vi "Create_Raw_data_file.vi"(4 "No of averages":i32=1, 5 "End time":dbl, 6 "Start time":dbl, 7 "Setup filename":string) -> (0 "Error String":string, 1 "Values":string[][](array[string]), 2 "Header Comments":string[](array[string]), 3 "Column headers":string[](array[string]))   [LabVIEW 2010]
uses:
  Controls/Post_Process.ctl
  Globals/Preference_global.vi
  Globals/Meas_global.vi
  Globals/Constants_global.vi
  Globals/Trav_pos_global.vi
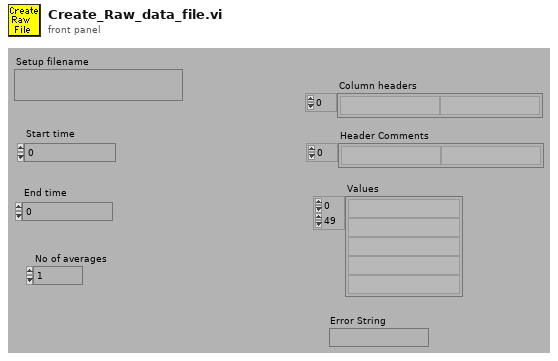
[diagram p1: front panel]
types:
  T1 = typedef "Post_Process.ctl" = enum16{"Take New Data", "Post Process Raw Data File"}
  T2 = typedef "Server_Comms.ctl" = enum16{"Server Link Healthy", "Do Not Link To Server"}
  T3 = typedef "Traverse_cluster.ctl" = cluster{"Start X":dbl, "Start Y":dbl, "Start Z":dbl, "End X":dbl, "End Y":dbl, "End Z":dbl, "No. of pts.":i32, "Spacing":T4, "Filename":path, "Tunnel Speed":dbl, "Averaging time (min)":dbl, "Extra Commands":string, "Specific Arguments":string, "Emission Rate (l/min)":dbl, "Trace Gas Concentration (%)":dbl, "Density Ratio":string, "Comments":string, "Row No":i32, "Row Type Selector":T5, "Completion time":string, "Row Duration (mins)":dbl, "No. of Valid pts.":i32, "Meas Setup File":string}
  T4 = typedef "Spacing.ctl" = enum16{"Linear", "Log", "Gauss", "Specified", "N/A"}
  T5 = typedef "Multi_run_mode.ctl" = enum16{"Move Traverse Only", "Set Tunnel Speed Only", "Set Source Only", "Set Measurement Conditions", "Single Measurement", "Vertical Profile", "Lateral Profile", "Longitudinal Profile", "Explore Volume", "Multi-Axis Profile", "Auto Calibrate", "Meas Fast FID Bkgnd", "Check Beam Power", "Scanning Valve Measurement", "Run VI Named:", "Set ADAM Ch", "Wait (minutes)", "Send Message", "Synchronize With:", "Fall Back to this Row", "Turn Off Row Repeating", "Blank Row"}
  T6 = cluster{"Name":string, "X":dbl, "Y":dbl, "Z":dbl}[]
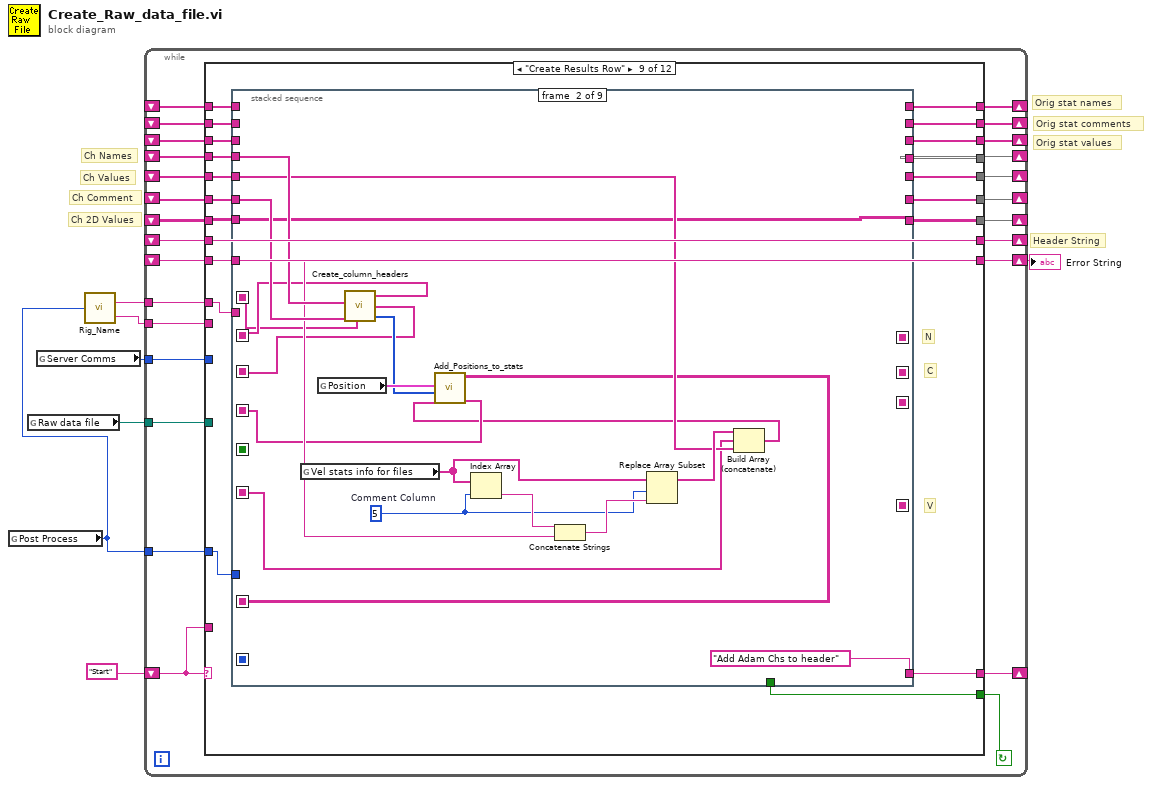
[diagram p0: block diagram]
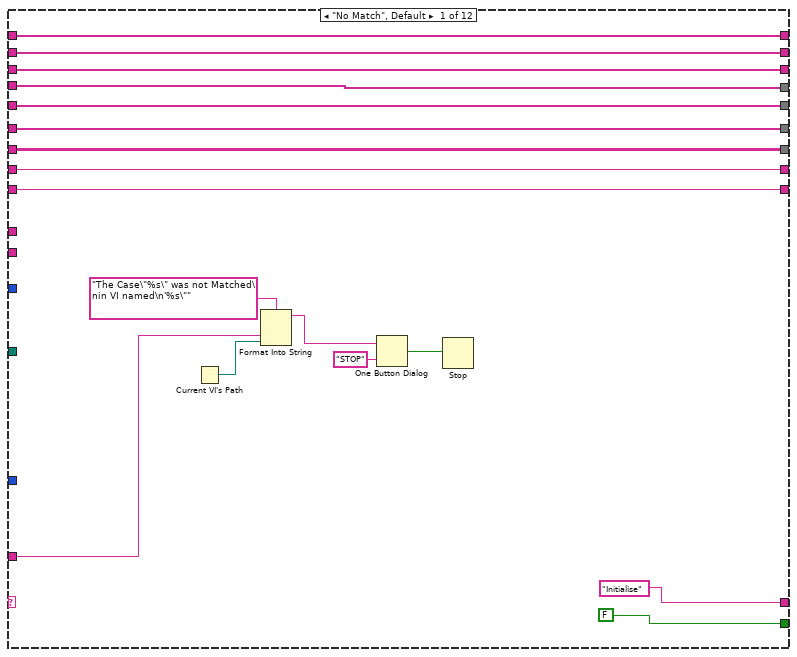
[diagram p2: hidden frame]
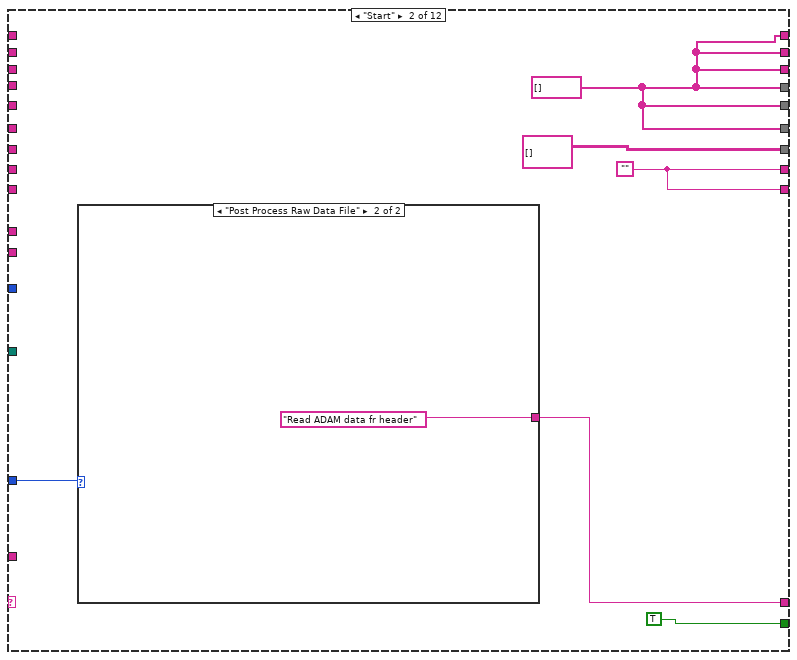
[diagram p3: hidden frame]
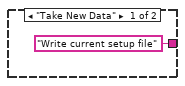
[diagram p4: hidden frame]
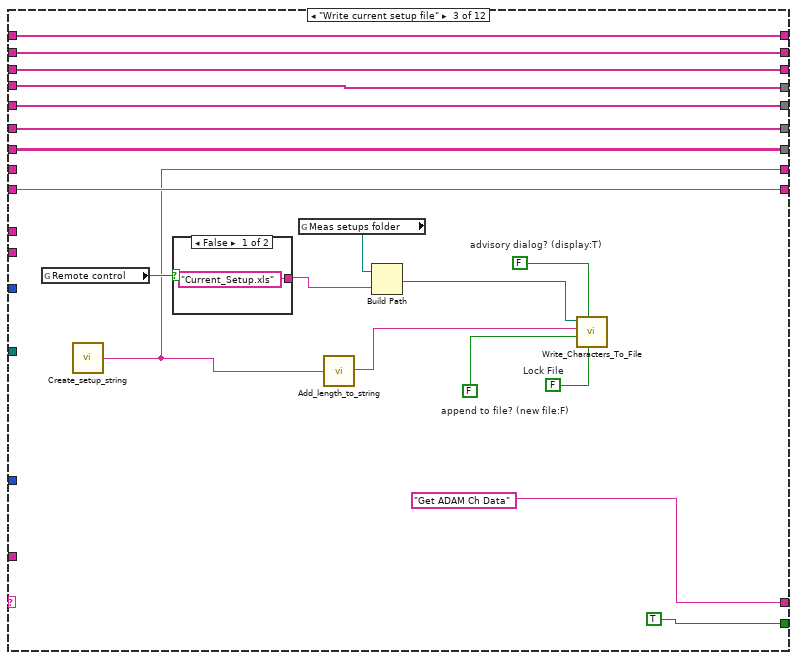
[diagram p5: hidden frame]
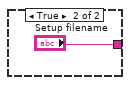
[diagram p6: hidden frame]
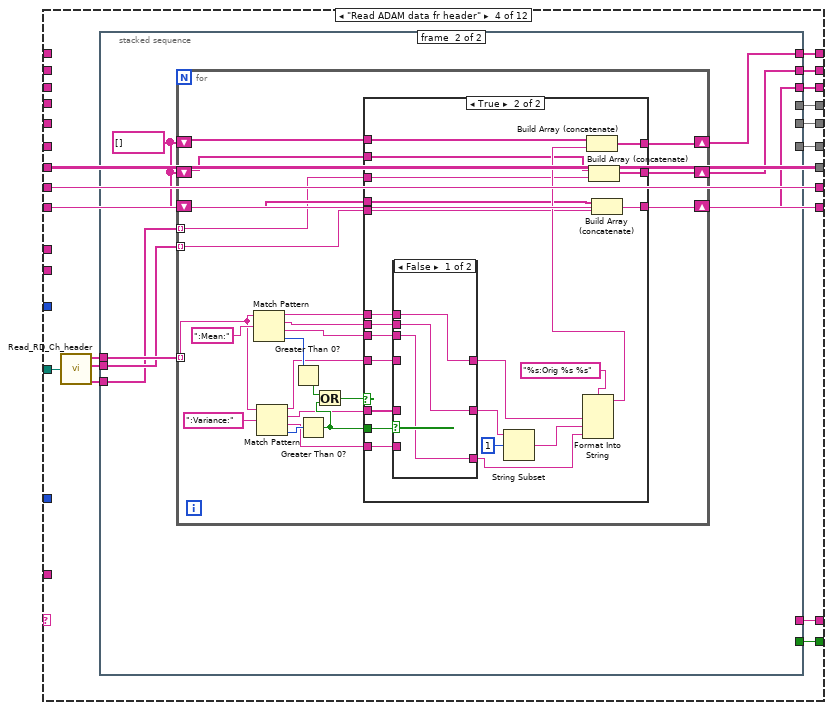
[diagram p7: hidden frame]
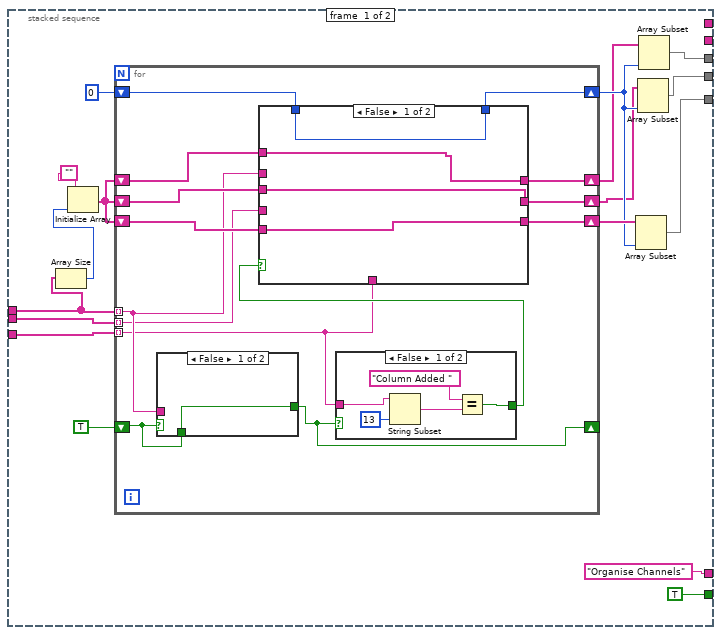
[diagram p8: hidden frame]
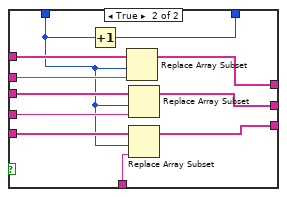
[diagram p9: hidden frame]
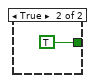
[diagram p10: hidden frame]
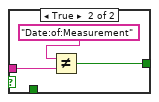
[diagram p11: hidden frame]
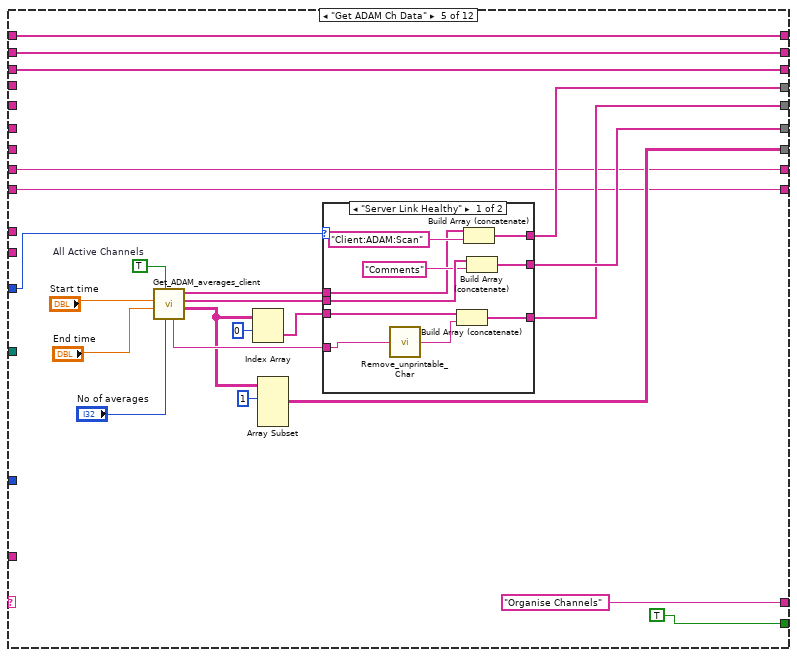
[diagram p14: hidden frame]
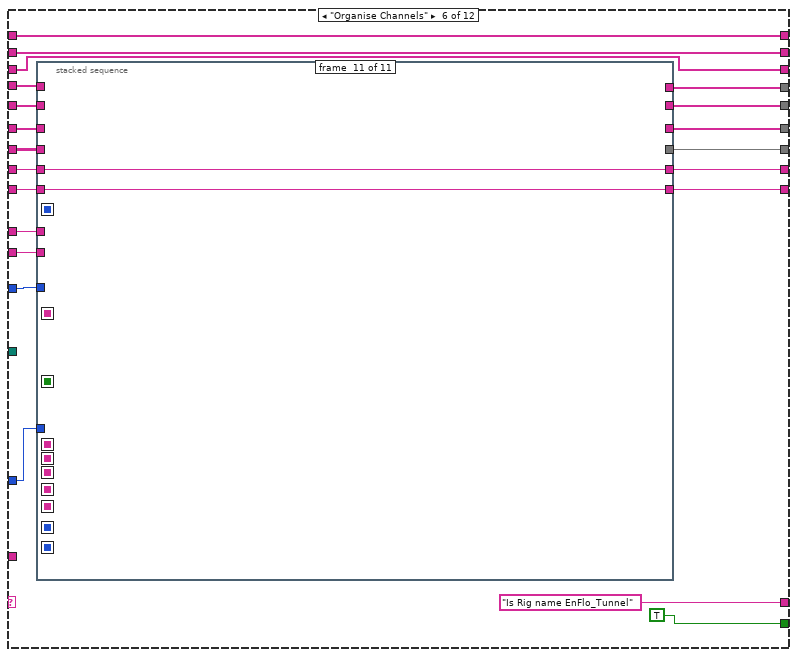
[diagram p16: hidden frame]
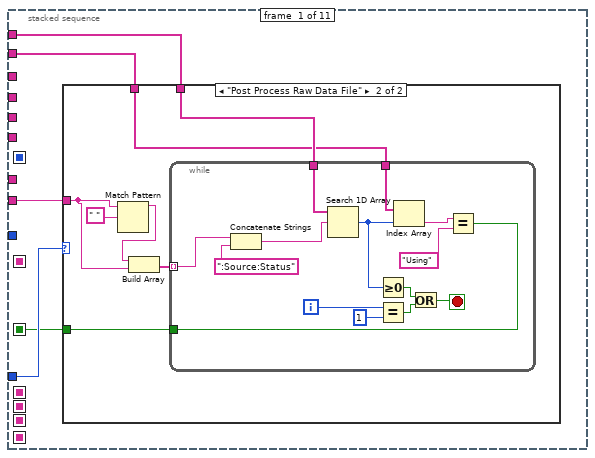
[diagram p17: hidden frame]
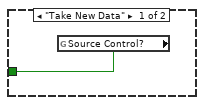
[diagram p18: hidden frame]
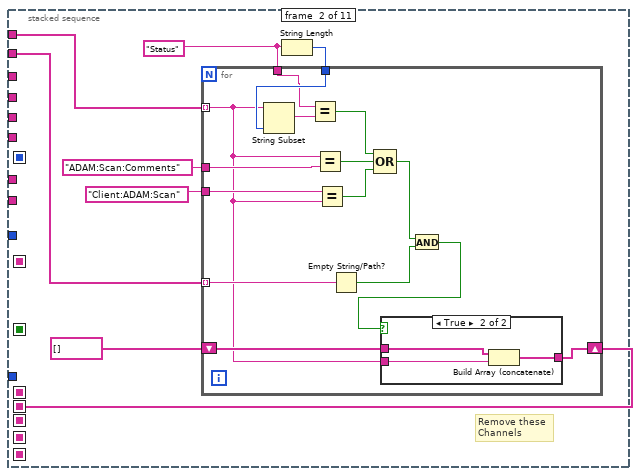
[diagram p19: hidden frame]
diagram:
  # "Orig stat values"
  # "Orig stat comments"
  # "Orig stat names"
  # "Header String"
  # "Ch 2D Values"
  # "Ch Comment"
  # "Ch Values"
  # "Ch Names"
  n1 = global read "Meas_global.vi" "Post Process"() -> (w3:T1)
  n2 = global read "Meas_global.vi" "Raw data file"() -> (w6:path)
  n3 = global read "Preference_global.vi" "Server Comms"() -> (w5:T2)
  n4 = call "Rig_Name.vi"("Post Process"=w3) -> ("Rig Setup before dash"=w2:string, "Hard Disk name"=w1:string)
  n5 = while {
    tunnel: w5 -> [w16]
    tunnel: w6 -> [w17]
    tunnel: w3 -> [w18]
    shift-left: _ -> [w20]
    shift-right: [w19] -> _
    shift-left: _ -> [w26]
    shift-right: [w25] -> w4
    shift-left: _ -> [w21]
    shift-right: [w27] -> _
    shift-left: _ -> [w22]
    shift-right: [w29] -> _
    shift-left: _ -> [w23]
    shift-right: [w28] -> _
    shift-left: _ -> [w24]
    shift-right: [w30] -> _
    shift-left: "Start" -> [w31]
    shift-right: [w32] -> _
    tunnel: w2 -> [w15]
    tunnel: w1 -> [w14]
    shift-right: [w10] -> _
    shift-left: _ -> [w11]
    shift-right: [w8] -> _
    shift-left: _ -> [w9]
    shift-right: [w12] -> _
    shift-left: _ -> [w13]
    stop <- w33 continue-if-true
    n6 = case shown="\"Create Results Row\"" w31 {
      tunnel: [FALSE TRUE TRUE w83 TRUE TRUE TRUE TRUE w604 TRUE TRUE FALSE] -> w33
      tunnel: ["Initialise" w52 "Get ADAM Ch Data" w94 "Organise Channels" "Is Rig name EnFlo_Tunnel" w541 "Create Results Row" w616 "Add Raw Data header info" "Add Raw Data fr Tempory file" "End"] -> w32
      tunnel: w31 -> [w45 _ _ _ _ _ _ _ _ _ _ _]
      tunnel: [w42 w51 w77 w85 w221 w264 w549 w559 w613 w884 w914 w931] -> w30
      tunnel: [w40 w51 w75 w86 w220 w260 w547 w557 w610 w895 w916 w933] -> w29
      tunnel: [w41 w51 w76 w84 w219 w261 w548 w558 w606 w896 w915 w932] -> w28
      tunnel: [w39 string[][] [] w74 w92 w217 w259 w546 w556 w608 w887 w917 w934] -> w27
      tunnel: w26 -> [w38 _ w72 w93 w216 w254 w543 w562 w614 w900 w918 w935]
      tunnel: [w38 w54 w72 w93 w216 w255 w543 w560 w614 w900 w918 w935] -> w25
      tunnel: w24 -> [w42 _ w77 _ _ w265 w549 w559 w612 w884 w914 w931]
      tunnel: w23 -> [w41 _ w76 _ _ w263 w548 w558 w607 w896 w915 w932]
      tunnel: w22 -> [w40 _ w75 _ _ w262 w547 w557 w611 w895 w916 w933]
      tunnel: w21 -> [w39 _ w74 w92 _ w258 w546 w556 w609 w887 w917 w934]
      tunnel: w20 -> [w37 _ _ w91 w215 w257 w544 w553 w615 w889 w911 w930]
      tunnel: [w37 w54 w63 w91 w215 w256 w544 w553 w615 w892 w910 ""] -> w19
      tunnel: w18 -> [_ w53 _ _ _ w250 _ _ w605 _ _ _]
      tunnel: w17 -> [_ _ _ w90 _ _ _ _ _ _ _ w926]
      tunnel: w16 -> [_ _ _ _ w214 w253 _ _ _ _ _ _]
      tunnel: w15 -> [_ _ _ _ _ w252 w538 _ w603 _ _ _]
      tunnel: w14 -> [_ _ _ _ _ w251 _ _ _ _ _ _]
      tunnel: w13 -> [w36 _ w61 _ w213 w249 w536 w552 w601 w881 w909 w923]
      tunnel: [w36 w51 w61 w82 w213 w249 w536 w552 w602 w881 w909 w923] -> w12
      tunnel: w11 -> [w35 _ w60 _ w212 w248 w535 w551 w600 w880 w908 w922]
      tunnel: [w35 w51 w60 w81 w212 w248 w535 w551 w599 w880 w908 w922] -> w10
      tunnel: w9 -> [w34 _ w59 _ w211 w247 w534 w550 w597 w879 w907 w921]
      tunnel: [w34 w51 w59 w80 w211 w247 w534 w550 w598 w879 w907 w921] -> w8
      frame "No Match", Default {
        n7 = Current VI's Path() -> (path=w44:path)
        n8 = Format Into String(format string="The Case\"%s\" was not Matched\nin VI named\n'%s\"" ("Format String"), w45, w44) -> (resulting string=w48:string)  [unwired: 2 in, 1 out]
        n9 = One Button Dialog(message=w48, button name ("OK")="STOP") -> (true=w46:bool)
        n10 = Stop(stop? (T)=w46) -> ()
      }
      frame "Start" {
        w54 = ""
        w51 = string[] []
        n11 = case shown="\"Post Process Raw Data File\"" w53 {
          tunnel: ["Write current setup file" "Read ADAM data fr header"] -> w52
          frame "Take New Data" {
          }
          frame "Post Process Raw Data File" {
          }
        }
      }
      frame "Write current setup file" {
        w65 = FALSE  # Lock File
        w70 = FALSE  # advisory dialog? (display:T)
        w71 = FALSE  # append to file? (new file:F)
        n12 = global read "Meas_global.vi" "Remote control"() -> (w69:bool)
        n13 = call "Create_setup_string.vi"() -> ("Setup String"=w63:string)  [unwired: 1 out]
        n14 = case shown="False" w69 {
          tunnel: ["Current_Setup.xls" ("Setup filename") "Setup filename"] -> w66
          frame False {
          }
          frame True {
          }
        }
        n15 = global read "Constants_global.vi" "Meas setups folder"() -> (w67:path)
        n16 = call "Add_length_to_string.vi"("String in"=w63) -> ("String out"=w68:string)
        n17 = Build Path(base path=w67, name or relative path=w66) -> (appended path=w64:path)
        n18 = call "Write_Characters_To_File.vi"("file path (dialog if empty)"=w64, "advisory dialog? (display:T)"=w70, "character string"=w68, "append to file? (new file:F)"=w71, "Lock File"=w65) -> ()  [unwired: 4 out]
      }
      frame "Read ADAM data fr header" {
        n19 = call "Read_RD_Ch_header.vi"("Raw data file"=w90) -> ("Ch Name Out"=w88:string[], "Ch Values"=w87:string[], "Comments"=w89:string[])  [unwired: 1 out]
        n20 = stacked-sequence {
          tunnel: ["Organise Channels" _] -> w94
          tunnel: w89 -> [w109 w154]
          tunnel: w88 -> [w108 w157]
          tunnel: w87 -> [w103 w155]
          tunnel: [w100 _] -> w86
          tunnel: [w97 _] -> w85
          tunnel: [w96 _] -> w84
          tunnel: [TRUE _] -> w83
          tunnel: [_ w153] -> w82
          tunnel: [_ w152] -> w81
          tunnel: [_ w151] -> w80
          frame #0 {
            n21 = Array Size(array=w108) -> (size(s)=w106:i32)
            n22 = Initialize Array("", w106) -> (w105:string[])
            n23 = for {
              shift-right: [w112] -> w101
              shift-left: 0 -> [w122]
              shift-right: [w116] -> w102
              shift-left: w105 -> [w119]
              shift-right: [w117] -> w99
              shift-left: w105 -> [w120]
              shift-right: [w118] -> w98
              shift-left: w105 -> [w121]
              shift-right: [w124] -> _
              shift-left: TRUE -> [w125]
              tunnel: w108 -> [w115] mode=indexing
              tunnel: w109 -> [w113] mode=indexing
              tunnel: w103 -> [w114] mode=indexing
              n24 = case shown="False" w125 {
                tunnel: w115 -> [_ w150]
                tunnel: [w147 w148] -> w124
                tunnel: w125 -> [w147 _]
                frame False {
                }
                frame True {
                  n25 = Not Equal?(x="Date:of:Measurement", y=w150) -> (x != y?=w148:bool)
                }
              }
              n26 = case shown="False" w124 {
                tunnel: w113 -> [w142 _]
                tunnel: [w144 TRUE] -> w123
                frame False {
                  n27 = String Subset(string=w142, length (rest)=13 ("length (rest)")) -> (substring=w141:string)  [unwired: 1 out]
                  n28 = Equal?(x="Column Added ", y=w141) -> (x = y?=w144:bool)
                }
                frame True {
                }
              }
              n29 = case shown="False" w123 {
                tunnel: w122 -> [w126 w131]
                tunnel: w121 -> [w129 w140]
                tunnel: w120 -> [w128 w139]
                tunnel: w119 -> [w127 w138]
                tunnel: [w129 w137] -> w118
                tunnel: [w128 w136] -> w117
                tunnel: [w127 w135] -> w116
                tunnel: w115 -> [_ w134]
                tunnel: w114 -> [_ w133]
                tunnel: w113 -> [_ w132]
                tunnel: [w126 w130] -> w112
                frame False {
                }
                frame True {
                  n30 = Increment(x=w131) -> (x+1=w130:i32)
                  n31 = Replace Array Subset(array=w140, new element=w134, index=w131) -> (w137:string[])
                  n32 = Replace Array Subset(array=w139, new element=w133, index=w131) -> (w136:string[])
                  n33 = Replace Array Subset(array=w138, new element=w132, index=w131) -> (w135:string[])
                }
              }
            }
            n34 = Array Subset(array=w102, length=w101) -> (w100:string[])  [unwired: 1 in]
            n35 = Array Subset(array=w99, length=w101) -> (w96:string[])  [unwired: 1 in]
            n36 = Array Subset(array=w98, length=w101) -> (w97:string[])  [unwired: 1 in]
          }
          frame #1 {
            w156 = string[] []
            n37 = for {
              shift-right: [w165] -> w153
              shift-left: w156 -> [w164]
              shift-right: [w158] -> w152
              shift-left: w156 -> [w159]
              shift-right: [w161] -> w151
              shift-left: w156 -> [w162]
              tunnel: w157 -> [w177] mode=indexing
              tunnel: w155 -> [w163] mode=indexing
              tunnel: w154 -> [w160] mode=indexing
              n38 = Match Pattern(string=w177, regular expression=":Mean:") -> (before substring=w168:string, match substring=w167:string, after substring=w166:string, offset past match=w176:i32)  [unwired: 1 out]
              n39 = Match Pattern(string=w177, regular expression=":Variance:") -> (before substring=w171:string, match substring=w170:string, after substring=w169:string, offset past match=w175:i32)  [unwired: 1 out]
              n40 = Greater Than 0?(x=w176) -> (x > 0?=w174:bool)
              n41 = Greater Than 0?(x=w175) -> (x > 0?=w172:bool)
              n42 = Or(x=w174, y=w172) -> (x .or. y?=w173:bool)
              n43 = case shown="True" w173 {
                tunnel: w172 -> [_ w204]
                tunnel: w171 -> [_ w203]
                tunnel: w170 -> [_ w202]
                tunnel: w169 -> [_ w201]
                tunnel: w168 -> [_ w194]
                tunnel: w167 -> [_ w193]
                tunnel: w166 -> [_ w192]
                tunnel: [w182 w190] -> w165
                tunnel: w164 -> [w182 w189]
                tunnel: w163 -> [_ w188]
                tunnel: w162 -> [w180 w187]
                tunnel: [w180 w186] -> w161
                tunnel: w160 -> [_ w185]
                tunnel: w159 -> [w181 w184]
                tunnel: [w181 w183] -> w158
                frame False {
                }
                frame True {
                  n44 = case shown="False" w204 {
                    tunnel: w203 -> [_ w209]
                    tunnel: w202 -> [_ w210]
                    tunnel: w201 -> [_ w208]
                    tunnel: [w206 w210] -> w199
                    tunnel: [w207 w209] -> w196
                    tunnel: [w205 w208] -> w195
                    tunnel: w194 -> [w207 _]
                    tunnel: w193 -> [w206 _]
                    tunnel: w192 -> [w205 _]
                    frame False {
                    }
                    frame True {
                    }
                  }
                  n45 = String Subset(string=w199, offset (0)=1) -> (substring=w198:string)  [unwired: 1 out]
                  n46 = Format Into String(format string="%s:Orig %s %s", w196, w198, w195) -> (resulting string=w191:string)  [unwired: 2 in, 1 out]
                  n47 = Build Array (concatenate)(w189, w191) -> (w190:string[])
                  n48 = Build Array (concatenate)(w184, w185) -> (w183:string[])
                  n49 = Build Array (concatenate)(w187, w188) -> (w186:string[])
                }
              }
            }
          }
        }
      }
      frame "Get ADAM Ch Data" {
        w224 = TRUE  # All Active Channels
        n50 = call "Get_ADAM_averages_client.vi"("No of averages"="No of averages", "All Active Channels"=w224, "End time"="End time", "Start time"="Start time") -> ("Values"=w227:string[][], "Comments"=w230:string[], "Titles"=w229:string[], "Messages"=w231:string)  [unwired: 1 in, 3 out]
        n51 = Index Array(array=w227, index (row)=0 ("Index")) -> (element=w218:string[])  [unwired: 1 in]
        n52 = Array Subset(array=w227, index (row)=1 ("Array Index")) -> (w217:string[][])  [unwired: 3 in]
        n53 = case shown="\"Server Link Healthy\"" w214 {
          tunnel: w231 -> [w235 _]
          tunnel: w230 -> [w243 w245]
          tunnel: w229 -> [w240 w246]
          tunnel: [w239 w246] -> w221
          tunnel: [w238 w245] -> w220
          tunnel: [w237 w244] -> w219
          tunnel: w218 -> [w236 w244]
          frame "Server Link Healthy" {
            n54 = call "Remove_unprintable_Char.vi"("Input String"=w235) -> ("Output String"=w234:string)
            n55 = Build Array (concatenate)(w236, w234) -> (w237:string[])
            n56 = Build Array (concatenate)(w240, "Client:ADAM:Scan") -> (w239:string[])
            n57 = Build Array (concatenate)(w243, "Comments" ("Comments")) -> (w238:string[])
          }
          frame "Do Not Link To Server" {
          }
        }
      }
      frame "Organise Channels" {
        n58 = stacked-sequence {
          seq-local: [_ _ _ _ _ _ _ _ w469 _ _] -> [_ _ _ _ _ _ _ _ _ w522 _]
          seq-local: [_ _ _ _ _ _ _ w435 _ _ _] -> [_ _ _ _ _ _ _ _ w464 _ _]
          seq-local: [_ _ _ _ _ _ _ w439 _ _ _] -> [_ _ _ _ _ _ _ _ w465 _ _]
          seq-local: [_ _ _ w327 _ _ _ _ _ _ _] -> [_ _ _ _ _ _ _ w441 w458 _ _]
          seq-local: [_ _ _ _ w348 _ _ _ _ _ _] -> [_ _ _ _ _ _ _ _ w462 _ _]
          seq-local: [_ _ _ _ _ w383 _ _ _ _ _] -> [_ _ _ _ _ _ _ _ w461 _ _]
          seq-local: [_ _ w322 _ _ _ _ _ _ _ _] -> [_ _ _ _ _ w382 w411 _ _ _ _]
          seq-local: [_ _ _ _ _ _ w410 _ _ _ _] -> [_ _ _ _ _ _ _ _ w460 _ _]
          seq-local: [w268 _ _ _ _ _ _ _ _ _ _] -> [_ _ _ w326 w347 _ _ _ w459 _ _]
          seq-local: [_ w297 _ _ _ _ _ _ _ _ _] -> [_ _ _ _ _ _ _ _ w457 _ _]
          tunnel: w265 -> [w270 w302 _ _ w351 w386 w415 w442 w467 w521 _]
          tunnel: [_ _ _ _ _ _ _ _ _ w520 _] -> w264
          tunnel: w263 -> [w269 w299 _ _ _ _ _ _ _ w519 _]
          tunnel: w262 -> [_ _ _ _ _ _ _ _ _ w518 _]
          tunnel: [_ _ _ _ _ _ _ _ _ w517 _] -> w261
          tunnel: [_ _ _ _ _ _ _ _ _ w516 _] -> w260
          tunnel: [_ _ _ _ _ _ _ _ _ w513 _] -> w259
          tunnel: w258 -> [_ _ _ _ _ _ _ _ _ w515 _]
          tunnel: w257 -> [_ _ _ _ _ _ _ _ _ _ w533]
          tunnel: [_ _ _ _ _ _ _ _ _ _ w533] -> w256
          tunnel: [_ _ _ _ _ _ _ _ _ _ w532] -> w255
          tunnel: w254 -> [_ _ _ _ _ _ _ _ _ _ w532]
          tunnel: w253 -> [_ _ _ _ _ _ _ w440 _ _ _]
          tunnel: w252 -> [_ _ _ w330 w350 w385 _ _ w463 _ _]
          tunnel: w251 -> [w272 _ _ _ _ _ _ _ _ _ _]
          tunnel: w250 -> [w271 _ _ _ _ _ _ _ _ _ _]
          frame #0 {
            n59 = case shown="\"Post Process Raw Data File\"" w271 {
              tunnel: w272 -> [_ w275]
              tunnel: w270 -> [_ w280]
              tunnel: w269 -> [_ w279]
              tunnel: [w273 w278] -> w268
              frame "Take New Data" {
                n60 = global read "Trav_pos_global.vi" "Source Control?"() -> (w273:bool)
              }
              frame "Post Process Raw Data File" {
                n61 = Match Pattern(string=w275, regular expression=" ") -> (before substring=w276:string)  [unwired: 4 out]
                n62 = Build Array(w276, w275) -> (w274:string[])
                n63 = while {
                  tunnel: w280 -> [w292]
                  tunnel: w279 -> [w291]
                  tunnel: [w288] -> w278
                  tunnel: w274 -> [w287] mode=indexing
                  i -> [w285]
                  stop <- w281 stop-if-true
                  n64 = Concatenate Strings(w287, ":Source:Status" ("string")) -> (w293:string)
                  n65 = Search 1D Array(1D array=w292, element=w293) -> (index of element=w286:i32)  [unwired: 1 out]
                  n66 = Greater Or Equal To 0?(x=w286) -> (x >= 0?=w282:bool)
                  n67 = Equal?(x=w285, y=1) -> (x = y?=w283:bool)
                  n68 = Index Array(array=w291, index=w286) -> (element=w290:string)
                  n69 = Or(x=w282, y=w283) -> (x .or. y?=w281:bool)
                  n70 = Equal?(x=w290, y="Using") -> (x = y?=w288:bool)
                }
              }
            }
          }
          frame #1 {
            w300 = "Status"
            # "Remove these\nChannels"
            n71 = String Length(string=w300) -> (length=w301:i32)
            n72 = for {
              tunnel: w302 -> [w309] mode=indexing
              tunnel: w301 -> [w317]
              tunnel: w300 -> [w315]
              tunnel: w299 -> [w314] mode=indexing
              shift-right: [w312] -> w297
              shift-left: string[] [] -> [w313]
              tunnel: "ADAM:Scan:Comments" -> [w311]
              tunnel: "Client:ADAM:Scan" -> [w310]
              n73 = String Subset(string=w309, length (rest)=w317) -> (substring=w316:string)  [unwired: 1 out]
              n74 = Equal?(x=w315, y=w316) -> (x = y?=w308:bool)
              n75 = Equal?(x=w309, y=w311) -> (x = y?=w307:bool)
              n76 = Equal?(x=w310, y=w309) -> (x = y?=w306:bool)
              n77 = Empty String/Path?(string/path=w314) -> (empty?=w305:bool)
              n78 = Compound Arithmetic op=OR(w308, w307, w306) -> (w304:bool)
              n79 = And(x=w304, y=w305) -> (x .and. y?=w303:bool)
              n80 = case shown="True" w303 {
                tunnel: w313 -> [w318 w321]
                tunnel: w309 -> [_ w320]
                tunnel: [w318 w319] -> w312
                frame False {
                }
                frame True {
                  n81 = Build Array (concatenate)(w321, w320) -> (w319:string[])
                }
              }
            }
          }
          frame #2 {
            n82 = Build Array("EnFlo_Tunnel:Reference:Velocity", "EnFlo_Tunnel:Chilled Water:Supply", "EnFlo_Tunnel:Chilled Water:Motor Temp") -> (w322:string[])
          }
          frame #3 {
            n83 = case shown="\"EnFlo_Tunnel\"" w330 {
              tunnel: [string[] [] w344] -> w328
              frame "False", Default {
              }
              frame "EnFlo_Tunnel" {
                n84 = Build Array("EnFlo_Tunnel:Reference:Velocity", "EnFlo_Tunnel:Usonic Fixed:Velocity", "EnFlo_Tunnel:Usonic Mobile:Velocity") -> (w344:string[])
              }
            }
            n85 = case shown="True" w326 {
              tunnel: [string[] [] w332] -> w329
              frame False {
              }
              frame True {
                n86 = Build Array("GMU:Source:Meas Q", "GMU:Source:Meas Strength", "GMU:Source:Meas Density", "GMU:Source:Type", "GMU:Release:Orientation", "GMU:Source:Height", "GMU:Trace:Gas", "GMU:Carrier 1:Gas", "GMU:Carrier 2:Gas") -> (w332:string[])
              }
            }
            n87 = Build Array (concatenate)(w328, w329) -> (w327:string[])
          }
          frame #4 {
            # "Remove these\nChannels"
            n88 = for {
              tunnel: w351 -> [w352] mode=indexing
              tunnel: w350 -> [w364]
              shift-right: [w365] -> w348
              shift-left: string[] [] -> [w366]
              tunnel: w347 -> [w357]
              w363 = " Metadata:"
              w370 = ":User:Name"
              n89 = case shown="False" w357 {
                tunnel: [w373 FALSE] -> w353
                tunnel: w352 -> [w372 _]
                frame False {
                  n90 = String Subset(string=w372, length (rest)=4 ("length (rest)")) -> (substring=w375:string)  [unwired: 1 out]
                  n91 = Equal?(x=w375, y="GMU:" ("regular expression")) -> (x = y?=w373:bool)
                }
                frame True {
                }
              }
              n92 = Match Pattern(string=w352, regular expression=w370) -> (offset past match=w371:i32)  [unwired: 4 out]
              n93 = Concatenate Strings(w364, w370) -> (w369:string)
              n94 = Match Pattern(string=w352, regular expression=w363) -> (offset past match=w361:i32)  [unwired: 4 out]
              n95 = Concatenate Strings(w364, w363) -> (w362:string)
              n96 = Greater Or Equal To 0?(x=w371) -> (x >= 0?=w367:bool)
              n97 = Not Equal?(x=w352, y=w369) -> (x != y?=w368:bool)
              n98 = Greater Or Equal To 0?(x=w361) -> (x >= 0?=w358:bool)
              n99 = And(x=w367, y=w368) -> (x .and. y?=w356:bool)
              n100 = Match Pattern(string=w352, regular expression=w362) -> (offset past match=w360:i32)  [unwired: 4 out]
              n101 = Less Than 0?(x=w360) -> (x < 0?=w359:bool)
              n102 = And(x=w358, y=w359) -> (x .and. y?=w355:bool)
              n103 = Compound Arithmetic op=OR(w356, w355, w353) -> (w354:bool)
              n104 = case shown="True" w354 {
                tunnel: w366 -> [w378 w381]
                tunnel: w352 -> [_ w380]
                tunnel: [w378 w379] -> w365
                frame False {
                }
                frame True {
                  n105 = Build Array (concatenate)(w381, w380) -> (w379:string[])
                }
              }
            }
          }
          frame #5 {
            # "Remove these\nChannels"
            n106 = for {
              tunnel: w386 -> [w389] mode=indexing
              tunnel: w385 -> [w390]
              shift-right: [w391] -> w383
              shift-left: string[] [] -> [w392]
              tunnel: w382 -> [w388]
              n107 = case shown="\"EnFlo_Tunnel\"" w390 {
                tunnel: [w393 FALSE] -> w387
                tunnel: w389 -> [w396 _]
                tunnel: w388 -> [w397 _]
                frame "False", Default {
                  w399 = "EnFlo_Tunnel:"
                  n108 = for {
                    tunnel: w397 -> [w404] mode=indexing
                    tunnel: w396 -> [w403]
                    tunnel: [w402] -> w394 mode=indexing
                    n109 = Not Equal?(x=w403, y=w404) -> (x != y?=w402:bool)
                  }
                  n110 = String Length(string=w399) -> (length=w401:i32)
                  n111 = String Subset(string=w396, length (rest)=w401) -> (substring=w400:string)  [unwired: 1 out]
                  n112 = And Array Elements(Boolean array=w394) -> (logical AND=w395:bool)
                  n113 = Equal?(x=w400, y=w399) -> (x = y?=w398:bool)
                  n114 = Compound Arithmetic op=AND(w398, w395) -> (w393:bool)
                }
                frame "EnFlo_Tunnel" {
                }
              }
              n115 = case shown="True" w387 {
                tunnel: w392 -> [w406 w409]
                tunnel: w389 -> [_ w408]
                tunnel: [w406 w407] -> w391
                frame False {
                }
                frame True {
                  n116 = Build Array (concatenate)(w409, w408) -> (w407:string[])
                }
              }
            }
          }
          frame #6 {
            w412 = "Correlation:"
            # "Remove these\nChannels"
            n117 = String Length(string=w412) -> (length=w413:i32)
            n118 = for {
              tunnel: w415 -> [w420] mode=indexing
              shift-right: [w429] -> w410
              shift-left: string[] [] -> [w430]
              tunnel: w413 -> [w428]
              tunnel: w412 -> [w427]
              tunnel: w411 -> [_]
              n119 = String Subset(string=w420, length (rest)=6 ("length (rest)")) -> (substring=w419:string)  [unwired: 1 out]
              n120 = Match Pattern(string=w419, regular expression="Orig[12345]_") -> (offset past match=w417:i32)  [unwired: 4 out]
              n121 = Equal?(x="Comments::", y=w420) -> (x = y?=w424:bool)
              n122 = Greater Than 0?(x=w417) -> (x > 0?=w416:bool)
              n123 = String Subset(string=w420, length (rest)=w428) -> (substring=w426:string)  [unwired: 1 out]
              n124 = Equal?(x=w426, y=w427) -> (x = y?=w423:bool)
              n125 = Compound Arithmetic op=OR(w416, w424, w423) -> (w422:bool)
              n126 = case shown="True" w422 {
                tunnel: w430 -> [w431 w434]
                tunnel: w420 -> [_ w433]
                tunnel: [w431 w432] -> w429
                frame False {
                }
                frame True {
                  n127 = Build Array (concatenate)(w434, w433) -> (w432:string[])
                }
              }
            }
          }
          frame #7 {
            n128 = case shown="\"Server Link Healthy\"" w440 {
              tunnel: [w444 i32[] []] -> w437
              tunnel: [w443 3] -> w439
              frame "Server Link Healthy" {
                w443 = 3
                n129 = for {
                  N: w443 -> [_]
                  tunnel: [w445] -> w444 mode=indexing
                  i -> [w445]
                }
              }
              frame "Do Not Link To Server" {
              }
            }
            n130 = for {
              tunnel: w442 -> [w452]
              tunnel: w441 -> [w451] mode=indexing
              shift-right: [w449] -> w436
              shift-left: i32[] [] -> [w450]
              n131 = Search 1D Array(1D array=w452, element=w451) -> (index of element=w448:i32)  [unwired: 1 out]
              n132 = case shown="0, Default" w448 {
                tunnel: w450 -> [w455 w456]
                tunnel: [w454 w456] -> w449
                tunnel: w448 -> [w453 _]
                frame 0, Default {
                  n133 = Build Array (concatenate)(w455, w453) -> (w454:i32[])
                }
                frame -1 {
                }
              }
            }
            n134 = Build Array (concatenate)(w436, w437) -> (w435:i32[])
          }
          frame #8 {
            n135 = Array Subset(array=w467, index=w465) -> (w466:string[])  [unwired: 1 in]
            n136 = Build Array (concatenate)(w458, w457, w462, w461, w460) -> (w468:string[])
            n137 = for {
              tunnel: w463 -> [w484]
              tunnel: w466 -> [w482] mode=indexing
              tunnel: w468 -> [w483]
              shift-right: [w478] -> w471
              shift-left: w464 -> [w479]
              shift-right: [w477] -> w472
              shift-left: i32[] [] -> [w480]
              tunnel: w465 -> [w474]
              tunnel: w459 -> [w473]
              i -> [w476]
              n138 = Search 1D Array(1D array=w483, element=w482) -> (index of element=w481:i32)  [unwired: 1 out]
              n139 = Add(x=w476, y=w474) -> (x+y=w475:i32)
              n140 = case shown="-1" w481 {
                tunnel: w484 -> [_ w497]
                tunnel: w482 -> [_ w491]
                tunnel: w480 -> [w485 w493]
                tunnel: w479 -> [w486 w496]
                tunnel: [w486 w495] -> w478
                tunnel: w475 -> [_ w494]
                tunnel: [w485 w492] -> w477
                tunnel: w473 -> [_ w487]
                frame 0, Default {
                }
                frame -1 {
                  n141 = Match Pattern(string=w491, regular expression=w497) -> (offset past match=w490:i32)  [unwired: 4 out]
                  n142 = Greater Or Equal To 0?(x=w490) -> (x >= 0?=w489:bool)
                  n143 = case shown="True" w487 {
                    tunnel: w491 -> [_ w504]
                    tunnel: w489 -> [w498 w500]
                    tunnel: [w498 w499] -> w488
                    frame False {
                    }
                    frame True {
                      n144 = Match Pattern(string=w504, regular expression="GMU:Source") -> (offset past match=w502:i32)  [unwired: 4 out]
                      n145 = Greater Or Equal To 0?(x=w502) -> (x >= 0?=w501:bool)
                      n146 = Or(x=w500, y=w501) -> (x .or. y?=w499:bool)
                    }
                  }
                  n147 = case shown="True" w488 {
                    tunnel: w496 -> [w508 w509]
                    tunnel: [w507 w509] -> w495
                    tunnel: w494 -> [w506 w511]
                    tunnel: w493 -> [w505 w512]
                    tunnel: [w505 w510] -> w492
                    frame True {
                      n148 = Build Array (concatenate)(w508, w506) -> (w507:i32[])
                    }
                    frame False {
                      n149 = Build Array (concatenate)(w512, w511) -> (w510:i32[])
                    }
                  }
                }
              }
            }
            n150 = Build Array (concatenate)(w471, w472) -> (w469:i32[])
          }
          frame #9 {
            n151 = for {
              tunnel: w522 -> [w523] mode=indexing
              tunnel: [w531] -> w520 mode=indexing
              tunnel: [w530] -> w517 mode=indexing
              tunnel: [w529] -> w516 mode=indexing
              tunnel: w521 -> [w528]
              tunnel: w519 -> [w527]
              tunnel: w518 -> [w526]
              tunnel: w515 -> [w525]
              tunnel: [w524] -> w514 mode=indexing
              n152 = Index Array(array=w528, index=w523) -> (element=w531:string)
              n153 = Index Array(array=w527, index=w523) -> (element=w530:string)
              n154 = Index Array(array=w526, index=w523) -> (element=w529:string)
              n155 = Index Array(array=w525, index (col)=w523) -> (element=w524:string[])  [unwired: 1 in]
            }
            n156 = Transpose 2D Array(2D array=w514) -> (transposed array=w513:string[][])
          }
          frame #10 {
          }
        }
      }
      frame "Is Rig name EnFlo_Tunnel" {
        n157 = Equal?(x=w538, y="EnFlo_Tunnel") -> (x = y?=w542:bool)
        n158 = Select(t="Check if Condensation occuring", s=w542, f="Create Results Row") -> (s? t:f=w541:string)
      }
      frame "Check if Condensation occuring" {
        n159 = Build Array("EnFlo_Tunnel:Chilled Water:Motor Temp", "EnFlo Lab:Hygrometry:Dew Point temp", "EnFlo_Tunnel:Chilled Water:Supply") -> (w585:string[])
        n160 = for {
          tunnel: w559 -> [w596]
          tunnel: w585 -> [w595] mode=indexing
          tunnel: w558 -> [w594]
          tunnel: [w592] -> w586 mode=indexing
          tunnel: [w591] -> w584 mode=indexing
          tunnel: [w590] -> w577 mode=indexing
          n161 = Search 1D Array(1D array=w596, element=w595) -> (index of element=w592:i32)  [unwired: 1 out]
          n162 = Index Array(array=w594, index=w592) -> (element=w593:string)
          n163 = Fract/Exp String To Number(string=w593) -> (number=w591:dbl)  [unwired: 4 out]
          n164 = Not A Number/Path/Refnum?(number/path/refnum=w591) -> (NaN/Path/Refnum?=w590:bool)
        }
        n165 = Less Than 0?(x=w586) -> (x < 0?=w576:bool[])
        n166 = Build Array (concatenate)(w577, w576) -> (w575:bool[])
        n167 = Or Array Elements(Boolean array=w575) -> (logical OR=w571:bool)
        n168 = Index Array(array=w584, index=0 ("Index")) -> (element=w578:dbl)
        n169 = Index Array(array=w584, index=1 ("Index")) -> (element=w574:dbl)
        n170 = Index Array(array=w584, index=2 ("Index")) -> (element=w566:dbl)
        n171 = Add(x=w574, y=2.5) -> (x+y=w567:dbl)
        n172 = Greater?(x=w578, y=43.0) -> (0:w572:bool)
        n173 = Greater?(x=w567, y=w566) -> (0:w573:bool)
        n174 = Subtract(x=w567, y=w566) -> (x-y=w565:dbl)
        n175 = Format Into String(format string=" Chilled water is %.1f deg below Condensation threshold. " ("Format String"), w565) -> (resulting string=w563:string)  [unwired: 2 in, 1 out]
        n176 = And(x=w572, y=w573) -> (x .and. y?=w570:bool)
        n177 = Compound Arithmetic op=AND(w570, invert w571) -> (w569:bool)
        n178 = Select(t=w563, s=w569, f="") -> (s? t:f=w561:string)
        n179 = Concatenate Strings(w562, w561) -> (w560:string)
      }
      frame "Create Results Row" {
        # "V"
        # "C"
        # "N"
        n180 = stacked-sequence {
          seq-local: [_ w659 _ _ _ _ _ _ _] -> [_ _ w681 w722 _ _ _ _ _]
          seq-local: [_ w658 _ _ _ _ _ _ _] -> [_ _ w677 w721 _ _ _ _ _]
          seq-local: [_ w657 _ _ _ _ _ _ _] -> [_ _ w675 w720 _ _ _ _ _]
          seq-local: [_ w654 _ _ _ _ _ _ _] -> [_ _ _ _ w757 _ _ _ _]
          seq-local: [_ _ _ w719 _ _ _ _ _] -> [_ _ _ _ w759 _ _ _ _]
          seq-local: [w618 _ _ _ _ _ _ _ _] -> [_ w653 _ _ _ _ _ _ _]
          seq-local: [w617 _ _ _ _ _ _ _ _] -> [_ w652 _ _ _ _ _ _ _]
          seq-local: [_ _ _ w718 _ _ _ _ _] -> [_ _ _ _ _ _ w812 w850 _]
          seq-local: [_ _ _ w717 _ _ _ _ _] -> [_ _ _ _ _ _ _ w848 _]
          seq-local: [_ _ _ _ w756 _ _ _ _] -> [_ _ _ _ _ _ _ w847 _]
          seq-local: [_ _ _ _ _ w774 _ _ _] -> [_ _ _ _ _ _ w811 w851 _]
          seq-local: [_ _ _ _ _ _ w810 _ _] -> [_ _ _ _ _ _ _ w849 _]
          tunnel: [_ "Add Adam Chs to header" _ _ _ _ _ _ _] -> w616
          tunnel: w612 -> [_ w670 w679 _ _ w777 _ _ _]
          tunnel: w611 -> [_ w669 w680 _ _ _ _ _ _]
          tunnel: w614 -> [_ w661 _ _ _ _ _ _ _]
          tunnel: w607 -> [_ w660 w674 _ _ w776 _ _ _]
          tunnel: w609 -> [_ w656 _ _ _ _ _ _ _]
          tunnel: [_ _ w678 _ _ _ _ _ _] -> w613
          tunnel: [_ _ w676 _ _ _ _ _ _] -> w610
          tunnel: [_ w656 _ _ _ _ _ _ _] -> w608
          tunnel: [_ _ w673 _ _ _ _ _ _] -> w606
          tunnel: w605 -> [_ _ w672 w723 _ w784 _ _ _]
          tunnel: [_ _ _ _ _ w780 _ _ _] -> w604
          tunnel: w603 -> [_ _ _ _ _ w778 _ _ _]
          tunnel: [_ _ _ _ _ _ _ _ w878] -> w602
          tunnel: w601 -> [_ _ _ _ _ _ _ w845 w878]
          tunnel: w600 -> [_ _ _ _ _ _ _ w842 w877]
          tunnel: [_ _ _ _ _ _ _ _ w877] -> w599
          tunnel: [_ _ _ _ _ _ _ _ w876] -> w598
          tunnel: w597 -> [_ _ _ _ _ _ _ w839 w876]
          frame #0 {
            n181 = global read "Trav_pos_global.vi" "Current Row"() -> (w622:T3)
            n182 = Unbundle By Name(w622) -> ("Row Type Selector"=w621:T5, "Specific Arguments"=w620:string)
            n183 = case shown="\"Single Measurement\"" w621 {
              tunnel: w620 -> [_ w628]
              tunnel: string[] [] -> [w623 w626]
              tunnel: [w623 w625] -> w618
              tunnel: [w623 w624] -> w617
              frame "Move Traverse Only", Default {
              }
              frame "Single Measurement" {
                n184 = call "Get_array_values_fr_String.vi"("String Value"=w628) -> ("String array"=w627:string[])  [unwired: 1 out]
                n185 = for {
                  tunnel: w627 -> [w631] mode=indexing
                  shift-right: [w629] -> w624
                  shift-left: w626 -> [w630]
                  shift-right: [w632] -> w625
                  shift-left: w626 -> [w633]
                  n186 = Match Pattern(string=w631, regular expression=":") -> (after substring=w637:string)  [unwired: 4 out]
                  n187 = Match Pattern(string=w637, regular expression=":") -> (after substring=w635:string)  [unwired: 4 out]
                  n188 = Match Pattern(string=w635, regular expression="=") -> (offset past match=w634:i32)  [unwired: 4 out]
                  n189 = case shown="0, Default" w634 {
                    tunnel: w633 -> [w649 w651]
                    tunnel: [w648 w651] -> w632
                    tunnel: w631 -> [w644 _]
                    tunnel: w630 -> [w641 w650]
                    tunnel: [w640 w650] -> w629
                    frame 0, Default {
                      n190 = Match Pattern(string=w644, regular expression="=") -> (before substring=w646:string, after substring=w645:string)  [unwired: 3 out]
                      n191 = call <vilib>:"Trim Whitespace.vi"("string"=w646) -> ("trimmed string"=w643:string)  [unwired: 1 in]
                      n192 = Build Array (concatenate)(w649, w643) -> (w648:string[])
                      n193 = call <vilib>:"Trim Whitespace.vi"("string"=w645) -> ("trimmed string"=w642:string)  [unwired: 1 in]
                      n194 = Build Array (concatenate)(w641, w642) -> (w640:string[])
                    }
                    frame -1 {
                    }
                  }
                }
              }
            }
          }
          frame #1 {
            w662 = 5  # Comment Column
            n195 = global read "Meas_global.vi" "Vel stats info for files"() -> (w663:string[])
            n196 = global read "Meas_global.vi" "Position"() -> (w668:T6)
            n197 = call "Create_column_headers.vi"("ADAM Titles"=w670, "ADAM Comments"=w669, "Additional Channels"=w653) -> ("Column headers"=w659:string[], "Header Comments"=w658:string[], "No of stats columns"=w667:i32[])  [unwired: 2 out]
            n198 = Index Array(array=w663, index=w662) -> (element=w665:string)
            n199 = Concatenate Strings(w665, w661) -> (w666:string)
            n200 = Replace Array Subset(array=w663, new element=w666, index=w662) -> (w664:string[])
            n201 = Build Array (concatenate)(w664, w652, w660) -> (w655:string[])
            n202 = call "Add_Positions_to_stats.vi"("Data row"=w655, "No of stats columns"=w667, "Position"=w668) -> ("Data row with positions"=w657:string[], "row splitting"=w654:string[][])  [unwired: 1 in, 6 out]
          }
          frame #2 {
            n203 = case shown="\"Post Process Raw Data File\"" w672 {
              tunnel: w681 -> [w690 _]
              tunnel: w680 -> [w689 w715]
              tunnel: w679 -> [w688 w716]
              tunnel: [w687 w716] -> w678
              tunnel: w677 -> [w686 _]
              tunnel: [w685 w715] -> w676
              tunnel: w675 -> [w684 _]
              tunnel: w674 -> [w683 w714]
              tunnel: [w682 w714] -> w673
              frame "Take New Data" {
                n204 = for {
                  tunnel: w688 -> [w701]
                  tunnel: w690 -> [w697] mode=indexing
                  shift-right: [w698] -> w687
                  shift-left: w688 -> [w699]
                  shift-right: [w695] -> w685
                  shift-left: w689 -> [w696]
                  shift-right: [w692] -> w682
                  shift-left: w683 -> [w693]
                  tunnel: w686 -> [w694] mode=indexing
                  tunnel: w684 -> [w691] mode=indexing
                  n205 = Search 1D Array(1D array=w701, element=w697) -> (index of element=w700:i32)  [unwired: 1 out]
                  n206 = case shown="-1" w700 {
                    tunnel: w699 -> [w704 w713]
                    tunnel: [w704 w711] -> w698
                    tunnel: w697 -> [_ w712]
                    tunnel: w696 -> [w703 w710]
                    tunnel: [w703 w709] -> w695
                    tunnel: w694 -> [_ w708]
                    tunnel: w693 -> [w702 w706]
                    tunnel: [w702 w705] -> w692
                    tunnel: w691 -> [_ w707]
                    frame 0, Default {
                    }
                    frame -1 {
                      n207 = Build Array (concatenate)(w706, w707) -> (w705:string[])
                      n208 = Build Array (concatenate)(w713, w712) -> (w711:string[])
                      n209 = Build Array (concatenate)(w710, w708) -> (w709:string[])
                    }
                  }
                }
              }
              frame "Post Process Raw Data File" {
              }
            }
          }
          frame #3 {
            # "Values"
            # "Comments"
            # "Ch Names"
            n210 = case shown="\"Post Process Raw Data File\"" w723 {
              tunnel: [w726 w732] -> w718
              tunnel: w722 -> [w726 w733]
              tunnel: [w725 w731] -> w717
              tunnel: w721 -> [w725 w729]
              tunnel: [w724 w730] -> w719
              tunnel: w720 -> [w724 w728]
              frame "Take New Data" {
              }
              frame "Post Process Raw Data File" {
                w727 = string[] []
                n211 = for {
                  shift-right: [w741] -> w732
                  shift-left: w727 -> [w742]
                  shift-right: [w736] -> w731
                  shift-left: w727 -> [w739]
                  shift-right: [w737] -> w730
                  shift-left: w727 -> [w738]
                  tunnel: w733 -> [w740] mode=indexing
                  tunnel: w729 -> [w735] mode=indexing
                  tunnel: w728 -> [w734] mode=indexing
                  n212 = Search 1D Array(1D array=w742, element=w740) -> (index of element=w743:i32)  [unwired: 1 out]
                  n213 = case shown="-1" w743 {
                    tunnel: w742 -> [w746 w755]
                    tunnel: [w746 w754] -> w741
                    tunnel: w740 -> [_ w753]
                    tunnel: w739 -> [w745 w752]
                    tunnel: w738 -> [w744 w751]
                    tunnel: [w744 w750] -> w737
                    tunnel: [w745 w749] -> w736
                    tunnel: w735 -> [_ w748]
                    tunnel: w734 -> [_ w747]
                    frame 0, Default {
                    }
                    frame -1 {
                      n214 = Build Array (concatenate)(w755, w753) -> (w754:string[])
                      n215 = Build Array (concatenate)(w752, w748) -> (w749:string[])
                      n216 = Build Array (concatenate)(w751, w747) -> (w750:string[])
                    }
                  }
                }
              }
            }
          }
          frame #4 {
            n217 = Array Size(array=w757) -> (size(s)=w762:i32[])
            n218 = Index Array(array=w762, index=0) -> (element=w760:i32)
            n219 = Greater Than 0?(x=w760) -> (x > 0?=w758:bool)
            n220 = case shown="True" w758 {
              tunnel: w759 -> [w764 w768]
              tunnel: w757 -> [_ w766]
              tunnel: [w763 w765] -> w756
              frame False {
                n221 = Build Array(w764) -> (w763:string[][])
              }
              frame True {
                n222 = Search 1D Array(1D array=w768, element="Instrument_name_place_holder") -> (index of element=w767:i32)  [unwired: 1 out]
                n223 = for {
                  tunnel: w768 -> [w773]
                  tunnel: w767 -> [w772]
                  tunnel: w766 -> [w771] mode=indexing
                  tunnel: [w770] -> w765 mode=indexing
                  n224 = Replace Array Subset(array=w773, new element=w771, index=w772) -> (w770:string[])
                }
              }
            }
          }
          frame #5 {
            n225 = Equal?(x="EnFlo_Tunnel", y=w778) -> (x = y?=w775:bool)
            n226 = case shown="True" w775 {
              tunnel: w777 -> [_ w797]
              tunnel: w776 -> [_ w794]
              tunnel: [FALSE w788] -> w774
              frame False {
              }
              frame True {
                n227 = global read "Meas_global.vi" "Pre Setup String"() -> (w793:string)
                n228 = Search 1D Array(1D array=w797, element="EnFlo_Tunnel:Heater:Enable") -> (index of element=w795:i32)  [unwired: 1 out]
                n229 = call "Get_Characters_from_string.vi"("Input string"=w793, "Variable name"="Show_all_EnFlo_Tunnel_Columns") -> ("Status"=w791:enum16{"Char in string", "Char not in string"}, "Value"=w790:string)  [unwired: 1 in]
                n230 = case shown="\"Char in string\"" w791 {
                  tunnel: w790 -> [w800 _]
                  tunnel: [w798 TRUE] -> w787
                  frame "Char in string" {
                    n231 = Equal?(x=w800, y="TRUE") -> (x = y?=w799:bool)
                    n232 = Not(x=w799) -> (.not. x?=w798:bool)
                  }
                  frame "Char not in string" {
                  }
                }
                n233 = case shown="-1" w795 {
                  tunnel: w795 -> [w808 _]
                  tunnel: w794 -> [w807 _]
                  tunnel: [w803 FALSE] -> w789
                  frame 0, Default {
                    n234 = Index Array(array=w807, index=w808) -> (element=w806:string)
                    n235 = Fract/Exp String To Number(string=w806) -> (number=w805:dbl)  [unwired: 4 out]
                    n236 = Less?(x=w805, y=0.5) -> (x < y?=w803:bool)
                  }
                  frame -1 {
                  }
                }
                n237 = Select(t=w789, s=w787, f=FALSE) -> (s? t:f=w788:bool)
              }
            }
            n238 = global read "Trav_pos_global.vi" "Dummy Measurement?"() -> (w781:bool)
            n239 = Equal?(x=Post_Process."Take New Data" ("Post Process"), y=w784) -> (x = y?=w782:bool)
            n240 = Compound Arithmetic op=AND(invert w781, w782) -> (w780:bool)
          }
          frame #6 {
            n241 = case shown="True" w811 {
              tunnel: w812 -> [_ w818]
              tunnel: [i32[] [] w816] -> w810
              frame False {
              }
              frame True {
                w814 = string[] ["EnFlo_Tunnel:Inlet Heater:Temp", "EnFlo_Tunnel:Inlet Rake:Temp", "EnFlo_Tunnel:Trav Thermo:", "EnFlo_Tunnel:floor ", "EnFlo_Tunnel:roof ", "EnFlo_Tunnel:Side ", "EnFlo_Tunnel:Temp:Inlet", "EnFlo_Tunnel:Temp:Floor"] ("Column headers")
                # "Remove these\nChannels"
                # "Remaining\nChannels"
                n242 = for {
                  tunnel: w814 -> [w820] mode=indexing
                  tunnel: [w819] -> w815 mode=indexing
                  n243 = String Length(string=w820) -> (length=w819:i32)
                }
                n244 = for {
                  tunnel: w818 -> [w824] mode=indexing
                  shift-right: [w827] -> w816
                  shift-left: i32[] [] -> [w828]
                  tunnel: w815 -> [w825]
                  tunnel: w814 -> [w823]
                  i -> [w826]
                  n245 = for {
                    tunnel: w825 -> [w833] mode=indexing
                    tunnel: w824 -> [w832]
                    tunnel: w823 -> [w830] mode=indexing
                    tunnel: [w829] -> w822 mode=indexing
                    n246 = String Subset(string=w832, length (rest)=w833) -> (substring=w831:string)  [unwired: 1 out]
                    n247 = Equal?(x=w831, y=w830) -> (x = y?=w829:bool)
                  }
                  n248 = Or Array Elements(Boolean array=w822) -> (logical OR=w821:bool)
                  n249 = case shown="True" w821 {
                    tunnel: w828 -> [w836 w837]
                    tunnel: w826 -> [w835 _]
                    tunnel: [w834 w837] -> w827
                    frame False {
                      n250 = Build Array (concatenate)(w836, w835) -> (w834:i32[])
                    }
                    frame True {
                    }
                  }
                }
              }
            }
          }
          frame #7 {
            n251 = case shown="True" w851 {
              tunnel: w850 -> [w857 w864]
              tunnel: w849 -> [_ w859]
              tunnel: w848 -> [w856 w863]
              tunnel: [w857 w862] -> w846
              tunnel: [w856 w861] -> w843
              tunnel: w847 -> [w855 w860]
              tunnel: [w855 w858] -> w840
              frame False {
              }
              frame True {
                n252 = for {
                  tunnel: w860 -> [w867] mode=indexing
                  tunnel: w859 -> [w866]
                  tunnel: [w865] -> w858 mode=indexing
                  n253 = for {
                    tunnel: w867 -> [w869]
                    tunnel: w866 -> [w870] mode=indexing
                    tunnel: [w868] -> w865 mode=indexing
                    n254 = Index Array(array=w869, index=w870) -> (element=w868:string)
                  }
                }
                n255 = for {
                  tunnel: w864 -> [w875]
                  tunnel: w859 -> [w871] mode=indexing
                  tunnel: w863 -> [w874]
                  tunnel: [w873] -> w862 mode=indexing
                  tunnel: [w872] -> w861 mode=indexing
                  n256 = Index Array(array=w874, index=w871) -> (element=w872:string)
                  n257 = Index Array(array=w875, index=w871) -> (element=w873:string)
                }
              }
            }
            n258 = for {
              tunnel: w840 -> [w854] mode=indexing
              tunnel: w839 -> [w853]
              tunnel: [w852] -> w838 mode=indexing
              n259 = Build Array (concatenate)(w854, w853) -> (w852:string[])
            }
            "Values" <- w838
            n260 = Build Array (concatenate)(w846, w845) -> (→"Column headers":string[])
            n261 = Build Array (concatenate)(w843, w842) -> (→"Header Comments":string[])
          }
          frame #8 {
          }
        }
      }
      frame "Add Adam Chs to header" {
        w882 = FALSE  # Email On Error?
        n262 = call "Channel_name_checker.vi"("Email On Error?"=w882, "Channel names"=w884) -> ("Channel names Out"=w883:string[])  [unwired: 1 out]
        n263 = for {
          tunnel: w883 -> [w906] mode=indexing
          tunnel: [w905] -> w899 mode=indexing
          tunnel: [w904] -> w898 mode=indexing
          tunnel: [w903] -> w897 mode=indexing
          n264 = call "Split_Ch_name.vi"("Ch name"=w906) -> ("Top level"=w905:string, "Middle"=w904:string, "Low level"=w903:string)
        }
        n265 = Array To Spreadsheet String(array=w887, 3:"%s" ("format string")) -> (spreadsheet string=w885:string)  [unwired: 1 out]
        n266 = Build Array(w899, w898, w897, w896, w895) -> (w893:string[][])
        n267 = Array To Spreadsheet String(array=w893, 3:"%s" ("format string")) -> (spreadsheet string=w886:string)  [unwired: 1 out]
        n268 = Concatenate Strings(w886, w885, "***************************************" ("Substring"), "\r", w889) -> (w892:string)
      }
      frame "Add Raw Data header info" {
        n269 = String Length(string=w911) -> (length=w913:i32)
        n270 = call "Raw_Data_File_Start_text.vi"("Header length"=w913) -> ("Start String"=w912:string)
        n271 = Concatenate Strings(w912, w911) -> (w910:string)
      }
      frame "Add Raw Data fr Tempory file" {
        w924 = 0  # Start to copy file at:
        n272 = global read "Constants_global.vi" "Data Folder Local"() -> (w928:path)
        n273 = Build Path(base path=w928, name or relative path="Tempory_Raw_Data_File.xls") -> (appended path=w925:path)
        n274 = call "Piece_file_Copy.vi"("File Start String"=w930, "Start to copy file at:"=w924, "Source File"=w925, "Target File"=w926) -> ()  [unwired: 1 out]
      }
    }
  }
  "Error String" <- w4
